vi "Convert Error to String.vi"(11 "error in (no error)":errorcluster) -> (3 "Error (Logic)":string)   [LabVIEW 2025, in "I2C Bus Monitor.lvclass"]
uses:
  I2C Bus Monitor.lvclass
  I2C Bus Monitor.lvclass/I2C Bus Monitor.ctl
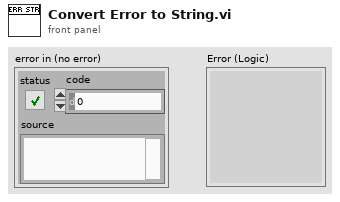
[diagram p1: front panel]
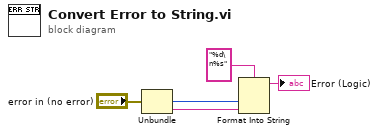
[diagram p0: block diagram]
diagram:
  n1 = Unbundle("error in (no error)") -> ("code"=w3:i32, "source"=w4:string)  [unwired: 1 out]
  n2 = Format Into String(format string="%d\n%s", w3, w4) -> (resulting string=→"Error (Logic)":string)  [unwired: 2 in, 1 out]
